vi "Initialize.vi"(8 "error in":errorcluster, 10 "resource":string, 11 "lia host in":refnum<class "LIA Host Interface RT.lvclass">) -> (0 "error out":errorcluster, 3 "lia host out":refnum<class "LIA Host Interface RT.lvclass">)   [LabVIEW 2017, in "LIA Host Interface RT.lvclass"]
uses:
  LIA Host Interface RT.lvclass
  Private/session data.ctl
  shared/Public/message.ctl
  LIA Host Interface RT.lvclass/LIA Host Interface RT.ctl
  shared/Lock-In Amplifier Example Shared.lvlib
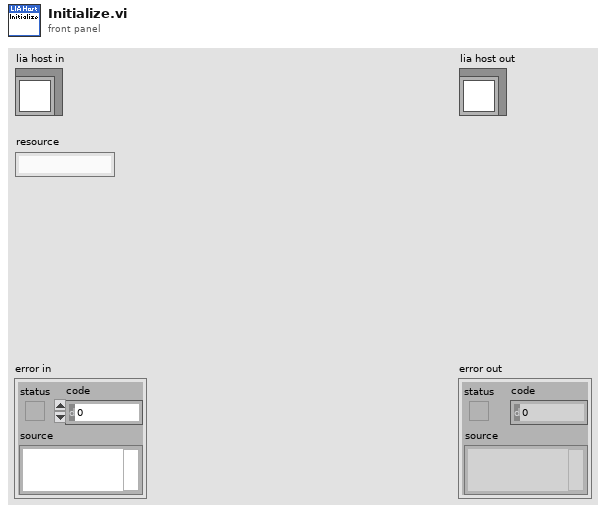
[diagram p1: front panel]
types:
  T1 = typedef "Lock-In Amplifier Example Shared.lvlib/message.ctl" = cluster{"command":u32, "payload":string}
  T2 = typedef "LIA Host Interface RT.lvclass/session data.ctl" = cluster{"tcp connection":refnum<k5>, "incoming data":refnum<queue>, "outgoing data":refnum<queue>, "lock-in data":refnum<queue>[], "stop process":refnum<notifier>}
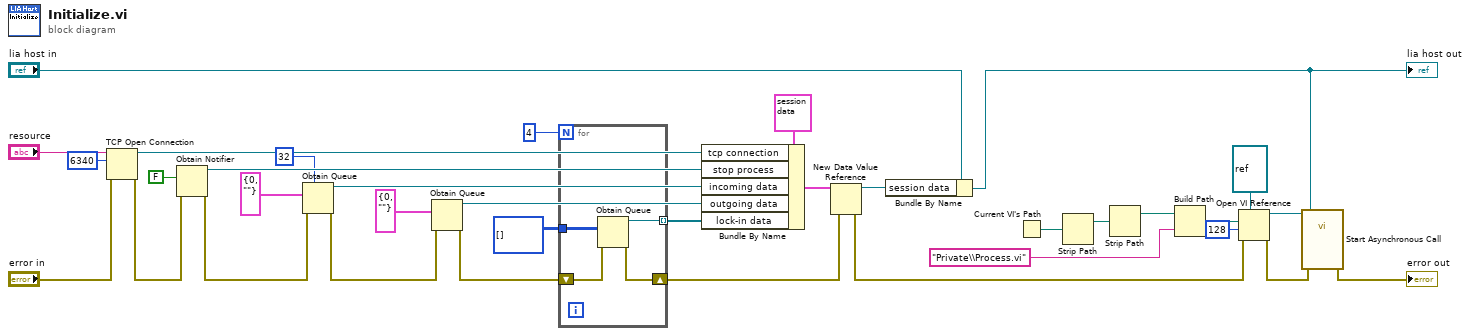
[diagram p0: block diagram]
diagram:
  n1 = TCP Open Connection(address="resource", remote port or service name=u16 6340, error in (no error)="error in") -> (connection ID=w28:refnum<k5>, error out=w33:errorcluster)  [unwired: 2 in]
  n2 = Obtain Notifier(notification data type=FALSE, error in (no error)=w33) -> (notifier out=w27:refnum<notifier>, error out=w31:errorcluster)  [unwired: 2 in, 1 out]
  n3 = Obtain Queue(max queue size (-1, unlimited)=32, element data type=T1 {"command"=0, "payload"=""}, error in (no error)=w31) -> (queue out=w26:refnum<queue>, error out=w10:errorcluster)  [unwired: 2 in, 1 out]
  n4 = Obtain Queue(element data type=T1 {"command"=0, "payload"=""}, error in (no error)=w10) -> (queue out=w8:refnum<queue>, error out=w9:errorcluster)  [unwired: 3 in, 1 out]
  n5 = for {
    N: 4 -> [_]
    shift-right: [w38] -> w24
    shift-left: w9 -> [w39]
    tunnel: i64[][] [] -> [w37]
    tunnel: [w36] -> w11 mode=indexing
    n6 = Obtain Queue(element data type=w37, error in (no error)=w39) -> (queue out=w36:refnum<queue>, error out=w38:errorcluster)  [unwired: 3 in, 1 out]
  }
  n7 = Bundle By Name(cluster=T2 {"tcp connection"=refnum, "incoming data"=refnum, "outgoing data"=refnum, "lock-in data"=[], "stop process"=refnum} ("session data"), "tcp connection"=w28, "stop process"=w27, "incoming data"=w26, "outgoing data"=w8, "lock-in data"=w11) -> (w25:T2)
  n8 = New Data Value Reference(data value=w25, error in=w24) -> (data value reference=w22:refnum<data-value>, error out=w21:errorcluster)
  n9 = Bundle By Name(cluster="lia host in", "session data"=w22) -> (w14:refnum<class "LIA Host Interface RT.lvclass">)
  "lia host out" <- w14
  n10 = Current VI's Path() -> (path=w20:path)
  n11 = Strip Path(path=w20) -> (stripped path=w4:path)  [unwired: 1 out]
  n12 = Strip Path(path=w4) -> (stripped path=w3:path)  [unwired: 1 out]
  n13 = Build Path(base path=w3, name or relative path="Private\\Process.vi") -> (appended path=w17:path)
  n14 = Open VI Reference(type specifier VI Refnum (for type only)=refnum<vi> refnum, vi path=w17, options=128, error in (no error)=w21) -> (vi reference=w15:refnum<vi>, error out=w13:errorcluster)  [unwired: 2 in]
  n15 = call-by-ref "Start Asynchronous Call"(reference=w15, error in=w13, "error in"=w13, "lia host in"=w14) -> (error out=→"error out":errorcluster)  [unwired: 8 in, 3 out]
